vi "Read Skip when tabbing.vi"(8 "error in (no error)":errorcluster, 11 "Bool D Element in":refnum<class "Bool D Element.lvclass">) -> (0 "error out":errorcluster, 2 "Skip when tabbing":bool, 3 "Bool D Element out":refnum<class "Bool D Element.lvclass">)   [LabVIEW 2018, in "D Datagrid Library.lvlib" / "Bool D Element.lvclass"]
uses:
  Bool D Element.lvclass
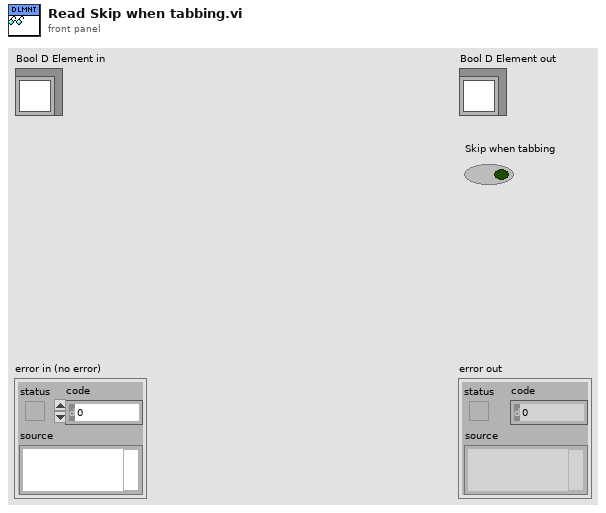
[diagram p1: front panel]
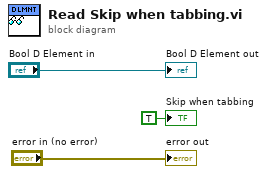
[diagram p0: block diagram]
diagram:
  "error out" <- "error in (no error)"
  "Bool D Element out" <- "Bool D Element in"
  "Skip when tabbing" <- TRUE ("Skip when tabbing")
